vi "GetAllDeviceKeys.vi"(8 "error in (no error)":errorcluster, 11 "USBLib In":refnum<k24>) -> (0 "error out":errorcluster, 1 "Device Keys Out":string[](array[string]), 2 "Device Count":i32, 3 "USBLib Out":refnum<k24>)   [LabVIEW 2009]
uses:
  C:/Samples/LabVIEW/UseDeviceKey/LabVIEW 2009/UseDeviceKey (with Device VIs)/UsbDllWrap.dll
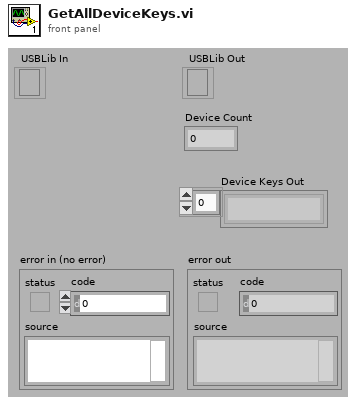
[diagram p1: front panel]
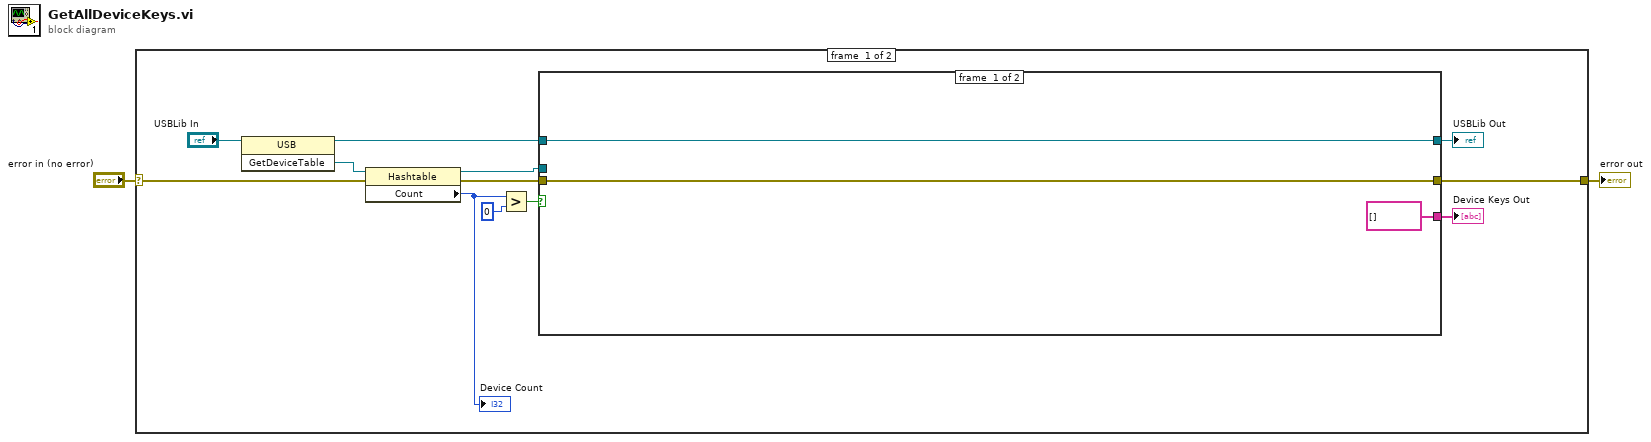
[diagram p0: block diagram]
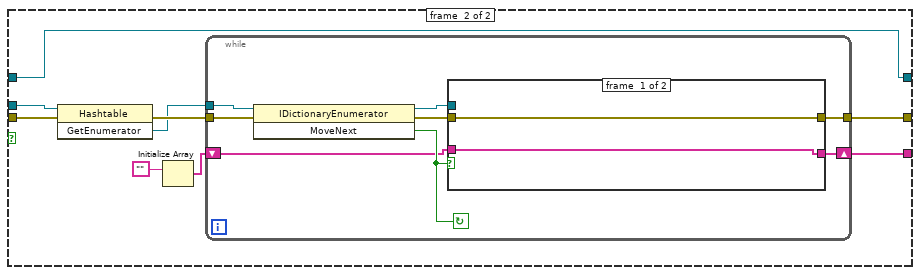
[diagram p2: hidden frame]
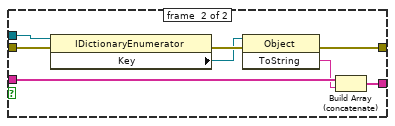
[diagram p3: hidden frame]
diagram:
  n1 = case shown="No Error" "error in (no error)" {
    selector: "error in (no error)" -> [w9 w45]
    tunnel: [w10 w45] -> w2
    frame #0 {
      n2 = invoke class="USB" method="GetDeviceTable"(reference="USBLib In") -> (reference out=w4:refnum<k24>, "GetDeviceTable"=w5:refnum<k24>)  [unwired: 2 in, 1 out]
      n3 = property class="Hashtable"(reference=w5, error in=w9) -> (reference out=w14:refnum<k24>, error out=w8:errorcluster, "Count"=w13:i32)
      "Device Count" <- w13
      n4 = Greater?(x=w13, y=0) -> (0:w11:bool)
      n5 = case shown="True" w11 {
        tunnel: w8 -> [w17 w26]
        tunnel: w14 -> [_ w19]
        tunnel: [w17 w23] -> w10
        tunnel: [string[] [] w21] -> w7
        tunnel: w4 -> [w16 w18]
        tunnel: [w16 w18] -> w3
        frame #0 {
        }
        frame #1 {
          n6 = invoke class="Hashtable" method="GetEnumerator"(reference=w19, error in=w26) -> (error out=w25:errorcluster, "GetEnumerator"=w24:refnum<k24>)  [unwired: 1 in, 1 out]
          n7 = Initialize Array("") -> (w20:string[])  [unwired: 1 in]
          n8 = while {
            tunnel: w25 -> [w34]
            tunnel: w24 -> [w33]
            tunnel: [w29] -> w23
            shift-right: [w28] -> w21
            shift-left: w20 -> [w27]
            stop <- w30 continue-if-true
            n9 = invoke class="IDictionaryEnumerator" method="MoveNext"(reference=w33, error in=w34) -> (reference out=w32:refnum<k24>, error out=w31:errorcluster, "MoveNext"=w30:bool)  [unwired: 1 in]
            n10 = case shown="False" w30 {
              tunnel: w32 -> [_ w44]
              tunnel: w31 -> [w36 w43]
              tunnel: [w36 w40] -> w29
              tunnel: w27 -> [w35 w39]
              tunnel: [w35 w37] -> w28
              frame #0 {
              }
              frame #1 {
                n11 = property class="IDictionaryEnumerator"(reference=w44, error in=w43) -> (error out=w42:errorcluster, "Key"=w41:refnum<k24>)  [unwired: 1 out]
                n12 = invoke class="Object" method="ToString"(reference=w41, error in=w42) -> (error out=w40:errorcluster, "ToString"=w38:string)  [unwired: 1 in, 1 out]
                n13 = Build Array (concatenate)(w39, w38) -> (w37:string[])
              }
            }
          }
        }
      }
      "USBLib Out" <- w3
      "Device Keys Out" <- w7
    }
    frame #1 {
    }
  }
  "error out" <- w2
